vi "DAQcardStorage.vi"(2 "error in":errorcluster, 3 "Channel Settings":T2(array[cluster]), 4 "Card Settings":T1(array[cluster]), 5 "Tree DVR In":refnum<data-value>) -> (0 "error out":errorcluster)   [LabVIEW 2014]
uses:
  <vilib>/MDSplus/Classes/Tree_Class/Tree.lvclass
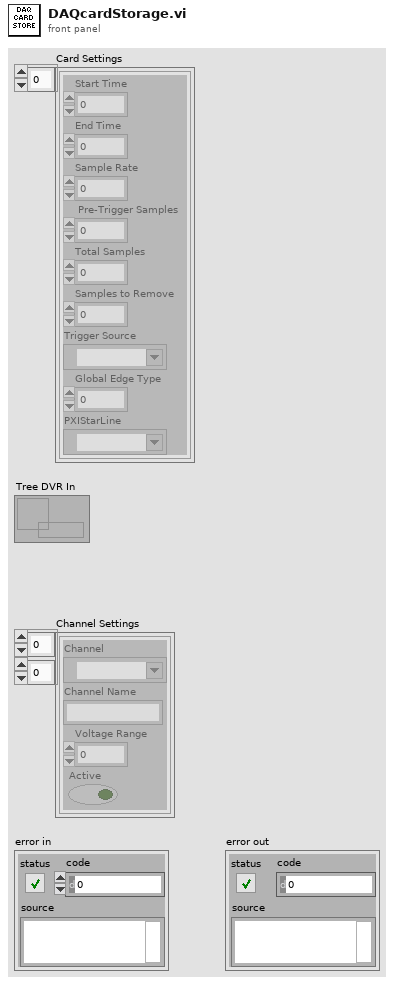
[diagram p1: front panel]
types:
  T1 = cluster{"Start Time":dbl, "End Time":dbl, "Sample Rate":dbl, " Pre-Trigger Samples":u32, "Total Samples":i32, "Samples to Remove":u32, "Trigger Source":tag, "Global Edge Type":i32, "PXIStarLine":tag}[]
  T2 = cluster{"Channel":tag, "Channel Name":string, "Voltage Range":dbl, "Active":bool}[][]
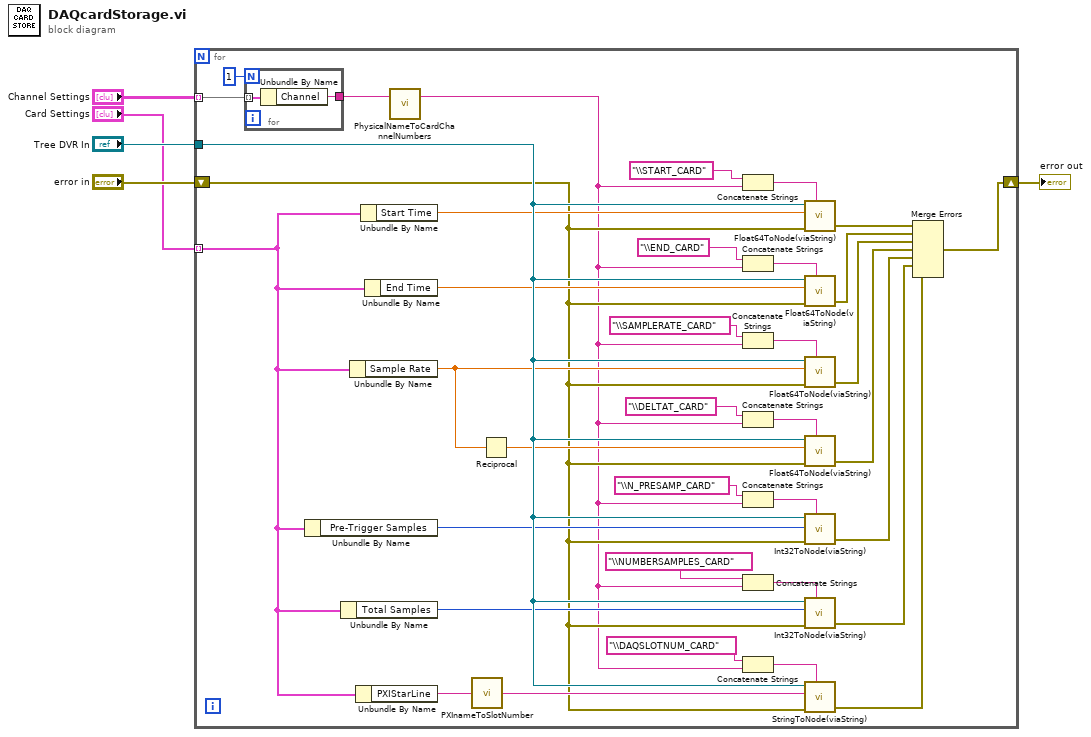
[diagram p0: block diagram]
diagram:
  n1 = for {
    tunnel: "Card Settings" -> [w42] mode=indexing
    tunnel: "Tree DVR In" -> [w41]
    shift-right: [w16] -> w2
    shift-left: "error in" -> [w15]
    tunnel: "Channel Settings" -> [w20] mode=indexing
    n2 = for {
      N: 1 -> [_]
      tunnel: w20 -> [w44] mode=indexing
      tunnel: [w43] -> w19
      n3 = Unbundle By Name(w44) -> ("Channel"=w43:tag)
    }
    n4 = Unbundle By Name(w42) -> ("Pre-Trigger Samples"=w31:u32)
    n5 = Unbundle By Name(w42) -> ("Total Samples"=w29:i32)
    n6 = Unbundle By Name(w42) -> ("Sample Rate"=w33:dbl)
    n7 = Unbundle By Name(w42) -> ("PXIStarLine"=w18:tag)
    n8 = Unbundle By Name(w42) -> ("Start Time"=w39:dbl)
    n9 = Unbundle By Name(w42) -> ("End Time"=w37:dbl)
    n10 = call "PhysicalNameToCardChannelNumbers.vi"("NI Physical Channel"=w19) -> ("Card #"=w7:string)  [unwired: 1 in, 1 out]
    n11 = call "PXInameToSlotNumber.vi"("PXI name"=w18) -> ("Slot #"=w17:string)
    n12 = Reciprocal(x=w33) -> (1/x=w34:dbl)
    n13 = Concatenate Strings("\\START_CARD" ("string"), w7) -> (w40:string)
    n14 = Concatenate Strings("\\END_CARD" ("string"), w7) -> (w38:string)
    n15 = Concatenate Strings("\\SAMPLERATE_CARD" ("string"), w7) -> (w36:string)
    n16 = Concatenate Strings("\\DELTAT_CARD" ("string"), w7) -> (w35:string)
    n17 = Concatenate Strings("\\N_PRESAMP_CARD" ("string"), w7) -> (w32:string)
    n18 = Concatenate Strings("\\NUMBERSAMPLES_CARD" ("string"), w7) -> (w30:string)
    n19 = Concatenate Strings("\\DAQSLOTNUM_CARD" ("string"), w7) -> (w28:string)
    n20 = call "Float64ToNode(viaString).vi"("Tree DVR in"=w41, "DBL in"=w39, "error in"=w15, "NodePath"=w40) -> ("error out"=w27:errorcluster)  [unwired: 1 in, 2 out]
    n21 = call "Float64ToNode(viaString).vi"("Tree DVR in"=w41, "DBL in"=w37, "error in"=w15, "NodePath"=w38) -> ("error out"=w26:errorcluster)  [unwired: 1 in, 2 out]
    n22 = call "Float64ToNode(viaString).vi"("Tree DVR in"=w41, "DBL in"=w33, "error in"=w15, "NodePath"=w36) -> ("error out"=w25:errorcluster)  [unwired: 1 in, 2 out]
    n23 = call "Float64ToNode(viaString).vi"("Tree DVR in"=w41, "DBL in"=w34, "error in"=w15, "NodePath"=w35) -> ("error out"=w24:errorcluster)  [unwired: 1 in, 2 out]
    n24 = call "Int32ToNode(viaString).vi"("Tree DVR in"=w41, "I32 in"=w31, "error in (no error)"=w15, "NodePath"=w32) -> ("error out"=w23:errorcluster)  [unwired: 1 in, 2 out]
    n25 = call "Int32ToNode(viaString).vi"("Tree DVR in"=w41, "I32 in"=w29, "error in (no error)"=w15, "NodePath"=w30) -> ("error out"=w22:errorcluster)  [unwired: 1 in, 2 out]
    n26 = call "StringToNode(viaString).vi"("Tree DVR in"=w41, "String value in"=w17, "error in (no error)"=w15, "NodePath"=w28) -> ("error out"=w21:errorcluster)  [unwired: 1 in, 2 out]
    n27 = Merge Errors(w27, w26, w25, w24, w23, w22, w21) -> (w16:errorcluster)
  }
  "error out" <- w2
